vi "振动测试client.vi"() -> ()   [LabVIEW 2010]
uses:
  <vilib>/Analysis/4window.llb/Hanning Window (DBL).vi
  <vilib>/Analysis/NI_AALPro.lvlib
  <vilib>/Analysis/NI_AALBase.lvlib
panel:
  in  "数据传输地址":string="dstp:\\\\10.10.22.19.wave"
  out "振动频率(Hz)":dbl=nan format="%.1f"
  out "加速度振幅\n(m/ss)":dbl=nan format="%.2f"
  in  "时\n    标":dbl(knob)=3.8811041886996547 scale=0.0..10.0 scale format="%.1f"
  in  "关闭":bool
  out "幅值频谱":cluster{dbl, "df":dbl, "Spectrum out":dbl[]}(graph)={0.0, "df"=nan, "Spectrum out"=[]}
  out "时域信号":cluster{i32, "时   标":dbl, dbl[][]}(graph)={0, "时   标"=3.8811041886996547, []}
  # "振 动 实 验 客 户 端"
  # "图例"
  # "Hz"
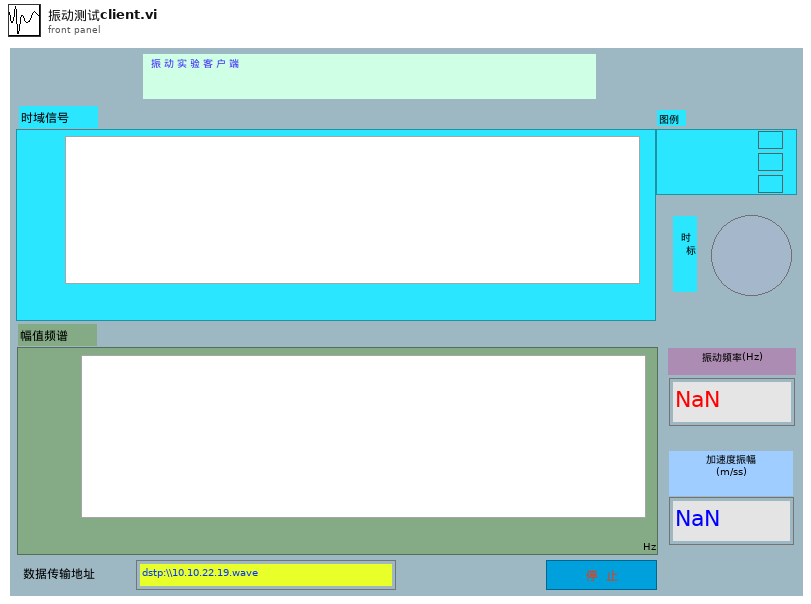
[diagram p1: front panel]
types:
  T1 = enum16{"Read", "Write", "ReadWrite", "BufferedRead", "BufferedReadWrite"}
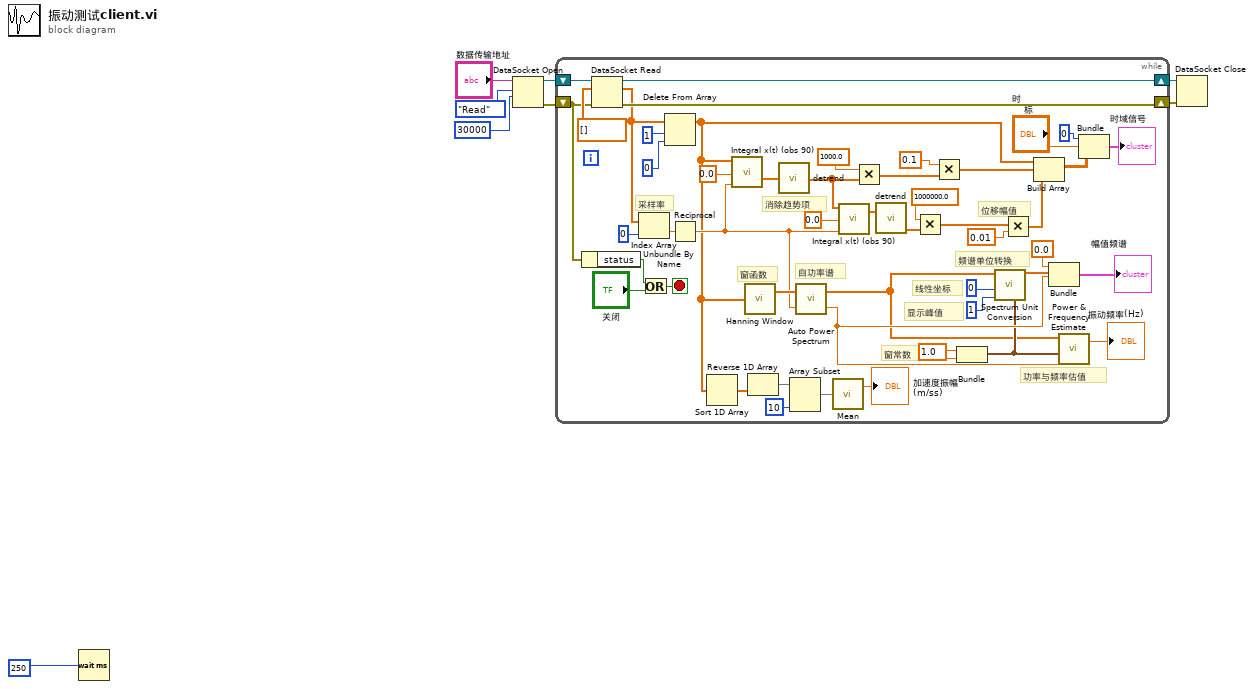
[diagram p0: block diagram]
diagram:
  n1 = Wait (ms)(milliseconds to wait=250) -> ()  [unwired: 1 out]
  n2 = DataSocket Open(9:30000 ("毫秒超时(10000)"), 10:T1."Read" ("模式"), 11:"数据传输地址") -> (0:w4:errorcluster, 3:w5:refnum<k13>)  [unwired: 1 in]
  n3 = while {
    shift-right: [w14] -> w6
    shift-left: w5 -> [w13]
    shift-right: [w28] -> w7
    shift-left: w4 -> [w11]
    stop <- w10 stop-if-true
    w35 = 1.0
    w57 = 0.0
    w46 = 0.0
    # "位移幅值"
    # "消除趋势项"
    # "窗函数"
    # "窗常数"
    # "自功率谱"
    # "线性坐标"
    # "显示峰值"
    # "频谱单位转换"
    # "功率与频率估值"
    # "采样率"
    n4 = Unbundle By Name(w11) -> ("status"=w9:bool)
    n5 = DataSocket Read(8:w11, 10:dbl[] [], 11:w13) -> (0:w28:errorcluster, 2:w23:dbl[], 3:w14:refnum<k13>)  [unwired: 2 in, 4 out]
    n6 = Index Array(array=w23, index=0 ("Index")) -> (element=w21:dbl)
    n7 = Or(x=w9, y="关闭") -> (x .or. y?=w10:bool)
    n8 = Delete From Array(array=w23, length=1, index=0) -> (array with subset deleted=w17:dbl[])  [unwired: 1 out]
    n9 = Reciprocal(x=w21) -> (1/x=w29:dbl)
    n10 = Sort 1D Array(array=w17) -> (sorted array=w16:dbl[])
    n11 = call <vilib>:"Integral x(t) (obs 90).vi"("dt"=w29, "final condition"=w46, "initial condition"=w46, "X"=w17) -> ("Integral X"=w53:dbl[])  [unwired: 1 out]
    n12 = call-poly <vilib>:"Hanning Window.vi"("X"=w17) -> ("Windowed X"=w30:dbl[])  [unwired: 1 out]
    n13 = Reverse 1D Array(array=w16) -> (reversed array=w18:dbl[])
    n14 = call "detrend.VI"("数据序列"=w53) -> ("处理后的数据序列"=w49:dbl[])
    n15 = Array Subset(array=w18, length=10) -> (w19:dbl[])  [unwired: 1 in]
    n16 = call <vilib>:"Auto Power Spectrum.vi"("dt"=w29, "Signal (V)"=w30) -> ("df"=w37:dbl, "Power Spectrum (V^2 rms)"=w33:dbl[])
    n17 = call <vilib>:"Mean.vi"("X"=w19) -> ("mean"=→"加速度振幅\n(m/ss)":dbl)  [unwired: 1 out]
    n18 = call <vilib>:"Integral x(t) (obs 90).vi"("dt"=w29, "final condition"=w57, "initial condition"=w57, "X"=w49) -> ("Integral X"=w54:dbl[])  [unwired: 1 out]
    n19 = Multiply(x=1000.0, y=w49) -> (x*y=w41:dbl[])
    n20 = call "detrend.VI"("数据序列"=w54) -> ("处理后的数据序列"=w45:dbl[])
    n21 = Multiply(x=1000000.0, y=w45) -> (x*y=w44:dbl[])
    n22 = Multiply(x=0.1, y=w41) -> (x*y=w52:dbl[])
    n23 = Bundle(w35, w35) -> (w36:cluster{dbl, dbl})  [unwired: 1 in]
    n24 = call <vilib>:"Spectrum Unit Conversion.vi"("window constants"=w36, "display unit"=1, "log/linear"=0, "Spectrum in"=w33) -> ("Spectrum out"=w32:dbl[])  [unwired: 6 in, 1 out]
    n25 = Multiply(x=w44, y=0.01) -> (x*y=w43:dbl[])
    n26 = Build Array(w17, w52, w43) -> (w51:dbl[][])
    n27 = Bundle(0.0, "df"=w37, "Spectrum out"=w32) -> (→"幅值频谱":cluster{dbl, "df":dbl, "Spectrum out":dbl[]})  [unwired: 1 in]
    n28 = call <vilib>:"Power & Frequency Estimate.vi"("df"=w37, "window constants"=w36, "Power Spectrum (V^2 rms)"=w33) -> ("est frequency peak"=→"振动频率(Hz)":dbl)  [unwired: 3 in, 1 out]
    n29 = Bundle(0, "时\n    标"="时\n    标", w51) -> (→"时域信号":cluster{i32, " \n 时\n    标":dbl, dbl[][]})  [unwired: 1 in]
  }
  n30 = DataSocket Close(8:w7, 11:w6) -> ()  [unwired: 1 in, 2 out]
